vi "SendRecieveFirebase.vi"() -> ()   [LabVIEW 2022 SP3]
uses:
  <vilib>/httpClient/PUTBuffer.vi
  <vilib>/httpClient/LabVIEWHTTPClient.lvlib
panel:
  out "String 2":string
  out "Cluster 2":T1
  out "String":string
  in  "Cluster":T1
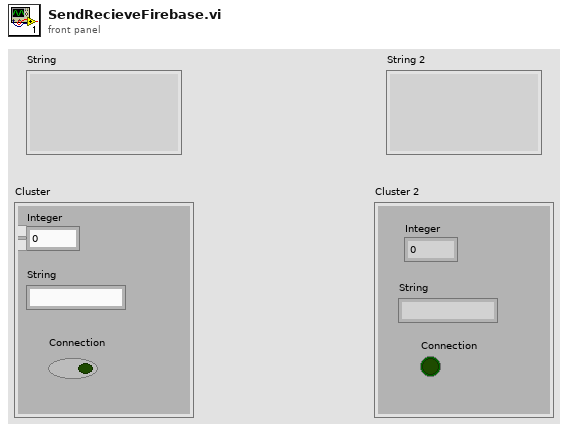
[diagram p1: front panel]
types:
  T1 = cluster{"Integer":dbl, "String":string, "Connection":bool}
  T2 = cluster{"Integer":i32, "String":string, "Connection":bool}
  T3 = typedef "LabVIEWHTTPClient.lvlib/ClientHandle.ctl" = refnum<k1>
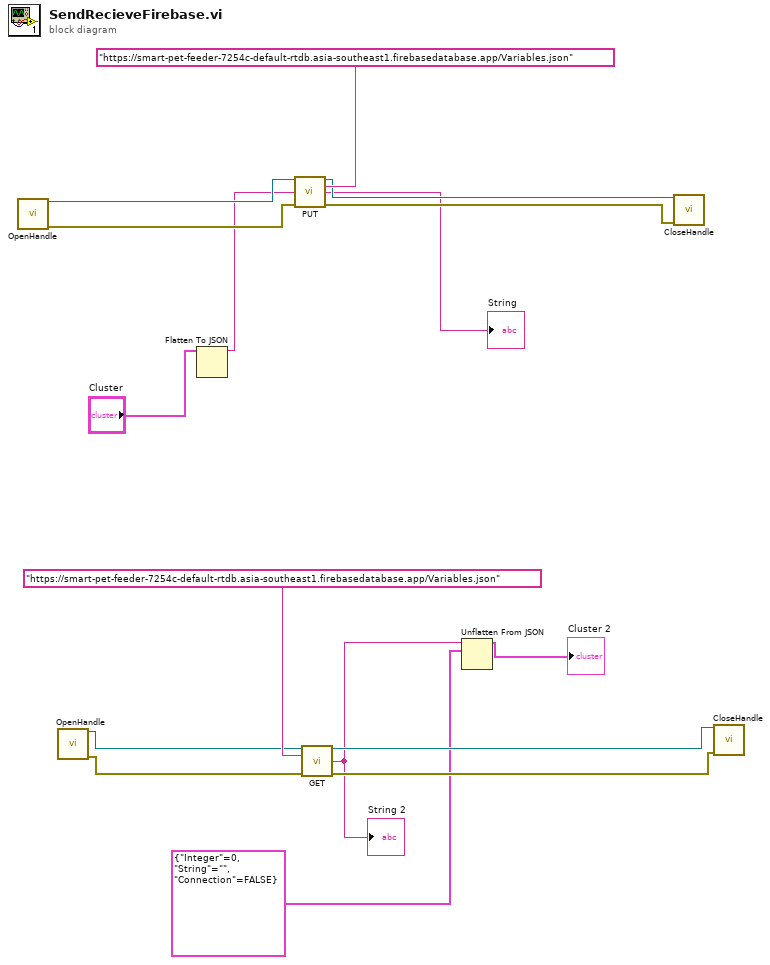
[diagram p0: block diagram]
diagram:
  n1 = call <vilib>:"OpenHandle.vi"() -> ("client handle out"=w15:T3, "error out"=w13:errorcluster)  [unwired: 14 in]
  n2 = call <vilib>:"OpenHandle.vi"() -> ("client handle out"=w7:T3, "error out"=w5:errorcluster)  [unwired: 14 in]
  n3 = Flatten To JSON(anything="Cluster") -> (JSON string=w10:string)  [unwired: 2 in, 1 out]
  n4 = call-poly <vilib>:"PUT.vi"("client handle"=w15, "url"="https://smart-pet-feeder-7254c-default-rtdb.asia-southeast1.firebasedatabase.app/Variables.json", "buffer"=w10, "error in (no error)"=w13) -> ("client handle out"=w14:T3, "body"=→"String":string, "error out"=w12:errorcluster)  [unwired: 8 in, 1 out]
  n5 = call <vilib>:"GET.vi"("client handle"=w7, "url"="https://smart-pet-feeder-7254c-default-rtdb.asia-southeast1.firebasedatabase.app/Variables.json", "error in (no error)"=w5) -> ("client handle out"=w6:T3, "body"=w3:string, "error out"=w4:errorcluster)  [unwired: 9 in, 1 out]
  "String 2" <- w3
  n6 = Unflatten From JSON(JSON string=w3, type and defaults=T2 {"Integer"=0, "String"="", "Connection"=FALSE}) -> (value=→"Cluster 2":T2)  [unwired: 5 in, 1 out]
  n7 = call <vilib>:"CloseHandle.vi"("client handle"=w14, "error in (no error)"=w12) -> ()  [unwired: 13 in, 1 out]
  n8 = call <vilib>:"CloseHandle.vi"("client handle"=w6, "error in (no error)"=w4) -> ()  [unwired: 13 in, 1 out]
